vi "json2csv.vi"() -> ()   [LabVIEW 2018]
uses:
  C:/Users/booko/Desktop/ENABLE/json2csv/bin/Debug/netstandard2.0/publish/CsvHelper.dll
  json2csv/bin/Debug/netstandard2.0/publish/CsvHelper.dll
  C:/Users/booko/Desktop/ENABLE/json2csv/bin/Debug/netstandard2.0/json2csv.dll
  json2csv/bin/Debug/netstandard2.0/json2csv.dll
  C:/Users/booko/Desktop/ENABLE/json2csv/bin/Debug/netstandard2.0/publish/Newtonsoft.Json.dll
  json2csv/bin/Debug/netstandard2.0/publish/Newtonsoft.Json.dll
panel:
  out "jsonToCSV":string
  in  "jsonContent":string="{\"x_Tx\":\"0,000\",\"y_Tx\":\"0,000\",\"z_Tx\":\"1,000\",\"th_Tx\":\"0,000\",\"phi_Tx\":\"0,000\",\"x_Rx\":\"0,000\",\"y_Rx\":\"0,000\",\"z_Rx\":\"1,000\",\"th_Rx\":\"0,000\",\"phi_Rx\":\"0,000\",\"f0\":\"2450000000,000\",\"BW\":\"20000000,000\",\"RX_custom_antenna\":\"\",\"TX_JX_custom_antenna\":\"\"}"
  in  "error in (no error)":errorcluster
  out "error out":errorcluster
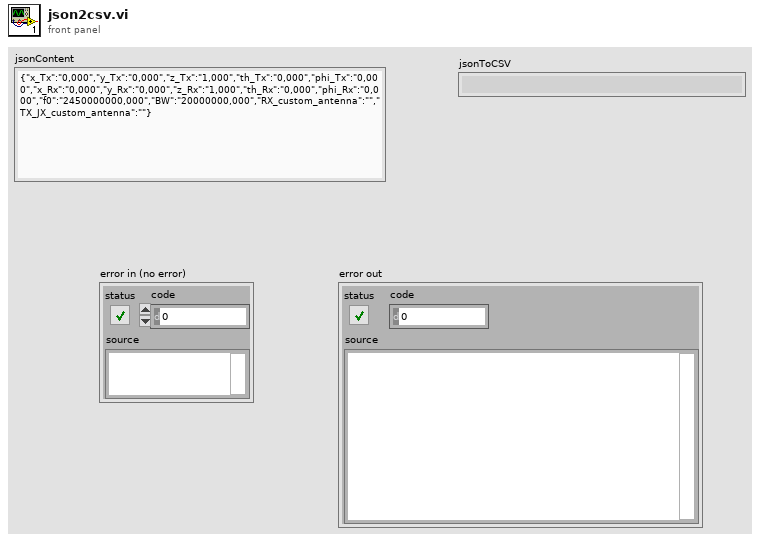
[diagram p1: front panel]
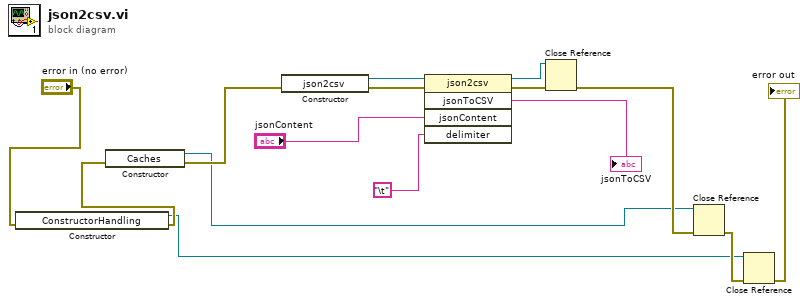
[diagram p0: block diagram]
diagram:
  n1 = constructor class="ConstructorHandling"(error in="error in (no error)") -> (reference out=w3:refnum<k24>, error out=w4:errorcluster)  [unwired: 2 in, 1 out]
  n2 = constructor class="Caches"(error in=w4) -> (reference out=w7:refnum<k24>, error out=w9:errorcluster)  [unwired: 2 in, 1 out]
  n3 = constructor class="json2csv"(error in=w9) -> (reference out=w15:refnum<k24>, error out=w13:errorcluster)  [unwired: 2 in, 1 out]
  n4 = invoke class="json2csv" method="jsonToCSV"(reference=w15, error in=w13, "jsonContent"="jsonContent", "delimiter"="\t") -> (reference out=w14:refnum<k24>, error out=w12:errorcluster, "jsonToCSV"=→"jsonToCSV":string)  [unwired: 1 in, 2 out]
  n5 = Close Reference(reference=w14, error in (no error)=w12) -> (error out=w8:errorcluster)
  n6 = Close Reference(reference=w7, error in (no error)=w8) -> (error out=w6:errorcluster)
  n7 = Close Reference(reference=w3, error in (no error)=w6) -> (error out=→"error out":errorcluster)
